vi "LVCAM Msg Receive.vi"(11 "LVCAM Msg Receive in":refnum<class "LVCAM Msg Receive.lvclass">) -> (0 "error out":errorcluster, 1 "DeQ Msg?":bool, 2 "Msg":refnum<class "Msg.lvclass">, 3 "LVCAM Msg Receive out":refnum<class "LVCAM Msg Receive.lvclass">)   [LabVIEW 2021, in "LVCAM.lvlib" / "LVCAM Msg Receive.lvclass"]
uses:
  LVCAM Msg Receive.lvclass
  Msg/Msg.lvclass
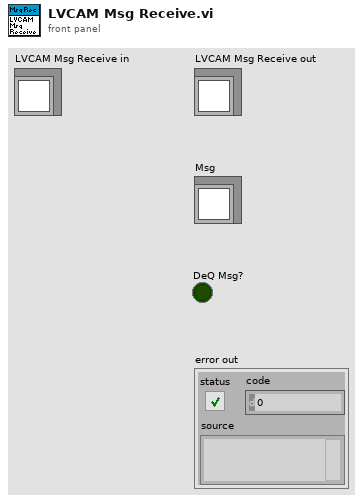
[diagram p1: front panel]
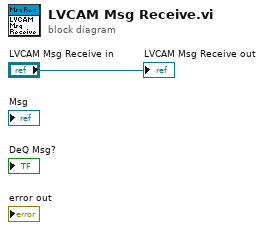
[diagram p0: block diagram]
diagram:
  "LVCAM Msg Receive out" <- "LVCAM Msg Receive in"
